vi "file_transfer_engine.vi"(10 "remote folder":string, 11 "Files to transfer BIN":path) -> ()   [LabVIEW 2017, in "labview-standard-library.lvlib"]
uses:
  labview-standard-library.lvlib
panel:
  in  "stop":bool
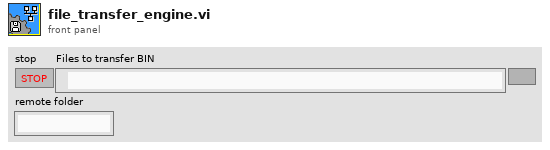
[diagram p1: front panel]
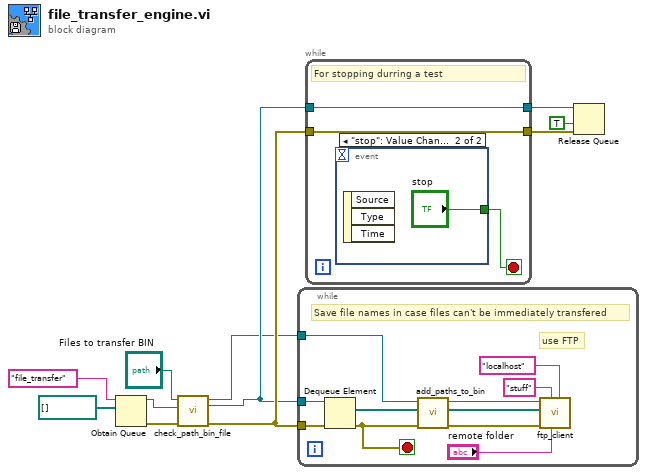
[diagram p0: block diagram]
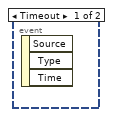
[diagram p2: hidden frame]
diagram:
  n1 = Obtain Queue(name (unnamed)="file_transfer", element data type=path[] []) -> (queue out=w3:refnum<queue>, error out=w6:errorcluster)  [unwired: 3 in, 1 out]
  n2 = call "check_path_bin_file.vi"("error in (no error)"=w6, "Queue in"=w3, "Files to transfer BIN in"="Files to transfer BIN") -> ("error out"=w5:errorcluster, "Queue out"=w2:refnum<queue>, "Files to transfer BIN refnum out"=w1:refnum<file>)  [unwired: 6 in]
  n3 = while {
    tunnel: w2 -> [w21]
    tunnel: w5 -> [w22]
    tunnel: w1 -> [w17]
    stop <- w18 stop-if-true
    # "use FTP"
    # "Save file names in case files can't be immediately transfered"
    n4 = Dequeue Element(queue=w21, error in (no error)=w22) -> (element=w14:path[], error out=w18:errorcluster)  [unwired: 1 in, 2 out]
    n5 = call "add_paths_to_bin.vi"("error in (no error)"=w18, "Files to transfer in"=w14, "Files to transfer bin file"=w17) -> ("error out"=w16:errorcluster, "Files to transfer out"=w13:path[], "path out"=w15:path)  [unwired: 6 in]
    n6 = call "ftp_client.vi"("Computer IP"="localhost", "remote folder"="remote folder", "password"="stuff", "error in (no error)"=w16, "Files to move"=w13, "files to transfer bin in"=w15) -> ()  [unwired: 6 in]
  }
  n7 = while {
    tunnel: w2 -> [w24]
    tunnel: [w24] -> w9
    tunnel: w5 -> [w23]
    tunnel: [w23] -> w7
    stop <- w25 stop-if-true
    # "For stopping durring a test"
    n8 = event shown="[1] \"stop\": Value Change" {
      selector: _ -> [_ _]
      dyn-events: _ -> [_ _]
      timeout: _ -> [_ _]
      tunnel: [_ "stop"] -> w25
      event Timeout {
        n9 = event-data() -> ()  [unwired: 1 in, 3 out]
      }
      event "stop": Value Change {
        n10 = event-data() -> ()  [unwired: 1 in, 3 out]
      }
    }
  }
  n11 = Release Queue(queue=w9, force destroy? (F)=TRUE, error in (no error)=w7) -> ()  [unwired: 3 out]
